vi "ReadSpec.vi"() -> (3 "其它规格":T1={"其它勾选类规格"={"保存图片"=FALSE, "上传设备状态数据"=FALSE, "保存数据"=FALSE, "开机默认开启监控摄像头"=FALSE, "启用mark拍照 "=FALSE}, "其它数据类规格"={"相机1像素-毫米换算系数"=15.0, "相机2像素-毫米换算系数"=15.0, "D盘剩余空间预警(G)"=15.0, "视频最长录制时间(秒)"=15.0}, "相机名称"={"相机1名称"="cam1", "相机2名称"="cam1", "Cam1启用"=FALSE, "Cam2启用"=FALSE, "Basler1"=FALSE, "Basler2"=FALSE}, "参数"={"Mark1曝光时间"=500, "Mark2曝光时间"=500, "二维码曝光时间"=500}} {"其它数据类规格"."视频最长录制时间(秒)" format="%.3f"; "其它数据类规格"."D盘剩余空间预警(G)" format="%.3f"; "其它数据类规格"."相机1像素-毫米换算系数" format="%.5f"; "其它数据类规格"."相机2像素-毫米换算系数" format="%.5f"})   [LabVIEW 2014]
uses:
  Controls/OtherSpec.ctl
  <vilib>/userdefined/High Color/IMAQdx.ctl
  Global.vi
  <vilib>/Utility/file.llb/Read From Spreadsheet File (string).vi
panel:
  out "all rows":string[][](array[string]) caption="所有行"
  out "数组":dbl[](array[numeric])
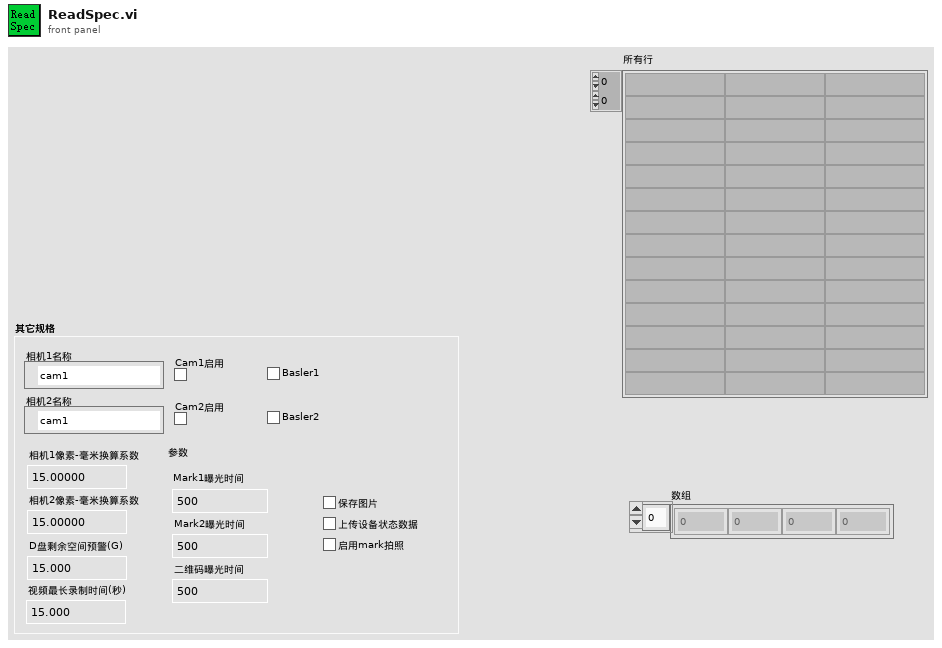
[diagram p1: front panel]
types:
  T1 = typedef "OtherSpec.ctl" = cluster{"其它勾选类规格":T2, "其它数据类规格":T3, "相机名称":T4, "参数":cluster{"Mark1曝光时间":i32, "Mark2曝光时间":i32, "二维码曝光时间":i32}}
  T2 = typedef "其它勾选类规格.ctl" = cluster{"保存图片":bool, "上传设备状态数据":bool, "保存数据":bool, "开机默认开启监控摄像头":bool, "启用mark拍照 ":bool}
  T3 = typedef "其他数据类规格.ctl" = cluster{"相机1像素-毫米换算系数":dbl, "相机2像素-毫米换算系数":dbl, "D盘剩余空间预警(G)":dbl, "视频最长录制时间(秒)":dbl}
  T4 = typedef "相机名称品牌使用状态.ctl" = cluster{"相机1名称":T5, "相机2名称":T5, "Cam1启用":bool, "Cam2启用":bool, "Basler1":bool, "Basler2":bool}
  T5 = typedef "IMAQdx.ctl" = refnum<k21>
  T6 = cluster{"[0]":bool, "[1]":bool, "[2]":bool, "[3]":bool, "[4]":bool}
  T7 = cluster{"[0]":dbl, "[1]":dbl, "[2]":dbl, "[3]":dbl}
  T8 = cluster{"String":string, "String":string, bool, bool, bool, bool}
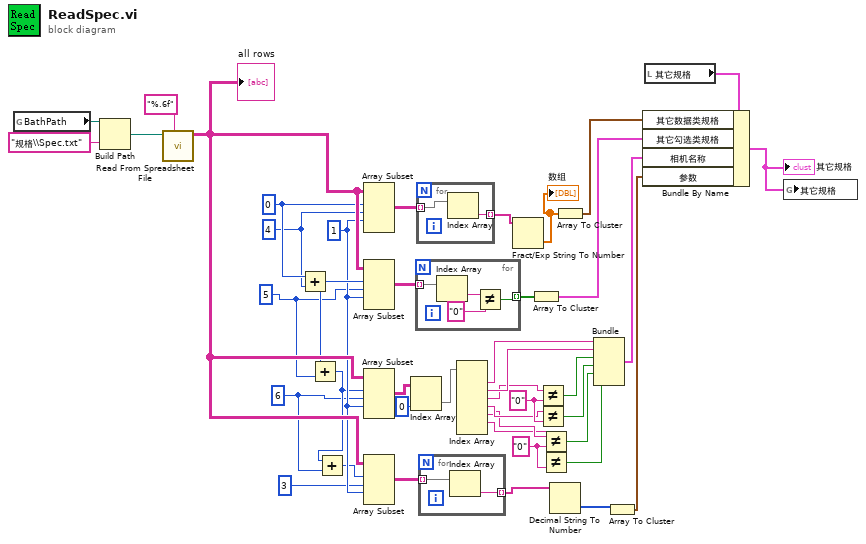
[diagram p0: block diagram]
diagram:
  w1 = 5
  w5 = 6 ("长度")
  w6 = 4
  w31 = "0" ("y")
  w32 = "0" ("y")
  w7 = 0 ("索引")
  w27 = 1 ("索引")
  n1 = global read "Global.vi" "BathPath"() -> (w42:path)
  n2 = Build Path(base path=w42, name or relative path="规格\\Spec.txt" ("名称或相对路径")) -> (appended path=w34:path)
  n3 = call-poly <vilib>:"Read From Spreadsheet File.vi"("format (%s)"="%.6f" ("format (%.3f)"), "file path (dialog if empty)"=w34) -> ("all rows"=w29:string[][])  [unwired: 5 in, 4 out]
  "all rows" <- w29
  n4 = Add(x=w7, y=w6) -> (x+y=w28:i32)
  n5 = Add(x=w28, y=w1) -> (x+y=w25:i32)
  n6 = Add(x=w25, y=w5) -> (x+y=w26:i32)
  n7 = Array Subset ("数组子集")(array=w29, index (row)=w7, length (row)=w6, index (col)=w27) -> (w40:string[][])  [unwired: 1 in]
  n8 = Array Subset ("数组子集")(array=w29, index (row)=w28, length (row)=w1, index (col)=w27) -> (w37:string[][])  [unwired: 1 in]
  n9 = Array Subset(array=w29, index (row)=w25, length (row)=w5, index (col)=w27) -> (w4:string[][])  [unwired: 1 in]
  n10 = Array Subset ("数组子集")(array=w29, index (row)=w26, length (row)=3 ("长度"), index (col)=w27) -> (w30:string[][])  [unwired: 1 in]
  n11 = Index Array(array=w4, index (col)=0 ("禁用的索引 (列)")) -> (element=w2:string[])  [unwired: 1 in]
  n12 = for {
    tunnel: w37 -> [w47] mode=indexing
    tunnel: [w44] -> w36 mode=indexing
    n13 = Index Array(array=w47) -> (element=w46:string)  [unwired: 1 in]
    n14 = Not Equal?(x=w46, y="0") -> (x != y?=w44:bool)
  }
  n15 = for {
    tunnel: w40 -> [w49] mode=indexing
    tunnel: [w48] -> w9 mode=indexing
    n16 = Index Array(array=w49) -> (element=w48:string)  [unwired: 1 in]
  }
  n17 = for {
    tunnel: w30 -> [w51] mode=indexing
    tunnel: [w50] -> w11 mode=indexing
    n18 = Index Array(array=w51) -> (element=w50:string)  [unwired: 1 in]
  }
  n19 = Index Array(array=w2) -> (element #1=w21:string, element #2=w20:string, element #3=w19:string, element #4=w18:string, element #5=w17:string, element #6=w16:string)  [unwired: 7 in, 1 out]
  n20 = Fract/Exp String To Number(string=w9) -> (number=w8:dbl[])  [unwired: 3 in, 1 out]
  "数组" <- w8
  n21 = Array To Cluster(array=w36) -> (cluster=w35:T6)
  n22 = Not Equal?(x=w19, y=w32) -> (x != y?=w15:bool)
  n23 = Not Equal?(x=w18, y=w32) -> (x != y?=w14:bool)
  n24 = Not Equal?(x=w17, y=w31) -> (x != y?=w13:bool)
  n25 = Not Equal?(x=w16, y=w31) -> (x != y?=w12:bool)
  n26 = Decimal String To Number(string=w11) -> (number=w10:i32[])  [unwired: 2 in, 1 out]
  n27 = Array To Cluster(array=w8) -> (cluster=w38:T7)
  n28 = Bundle("String"=w21, "String"=w20, w15, w14, w13, w12) -> (w22:T8)  [unwired: 1 in]
  n29 = Array To Cluster(array=w10) -> (cluster=w23:cluster{"[0]":i32, "[1]":i32, "[2]":i32})
  n30 = local read "其它规格"() -> (w39:T1)
  n31 = Bundle By Name(cluster=w39, "其它数据类规格"=w38, "其它勾选类规格"=w35, "相机名称"=w22, "参数"=w23) -> (w33:T1)
  "其它规格" <- w33
  n32 = global write "Global.vi" "其它规格"(w33) -> ()
